vi "TDMS Copy Channel Data.vi"(5 "channel name":string, 7 "group name":string, 8 "error in":errorcluster, 9 "Chunk Size (65536)":i64=65536 min=1, 10 "tdms dest in":refnum<k34>, 11 "tdms source in":refnum<k34>) -> (0 "error out":errorcluster, 2 "tdms dest out":refnum<k34>, 3 "tdms source out":refnum<k34>)   [LabVIEW 2011]
doc: "Copies the data from Channel in the source file to the destintion file. If the channel exists there, the data is appended to the old one."
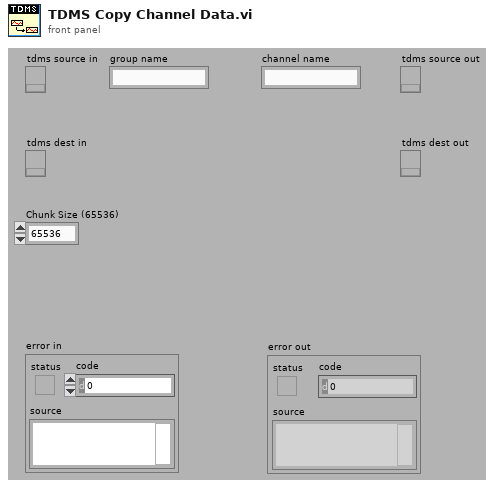
[diagram p1: front panel]
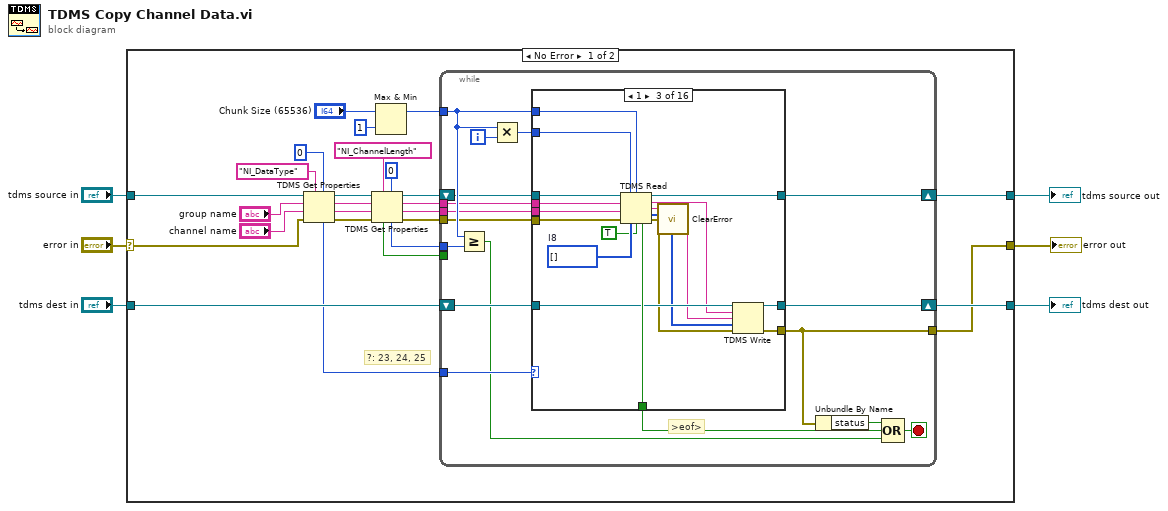
[diagram p0: block diagram]
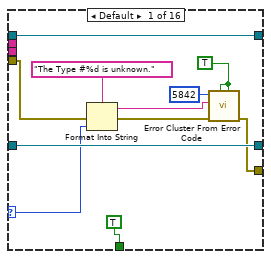
[diagram p2: hidden frame]
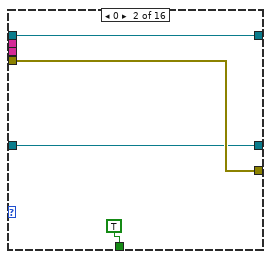
[diagram p3: hidden frame]
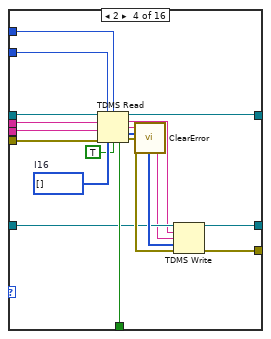
[diagram p4: hidden frame]
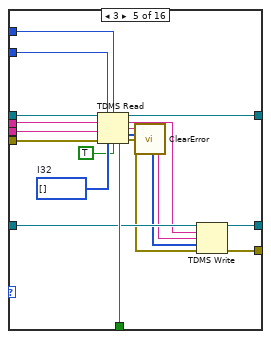
[diagram p5: hidden frame]
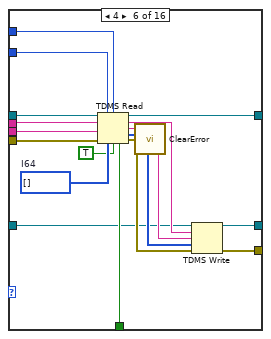
[diagram p6: hidden frame]
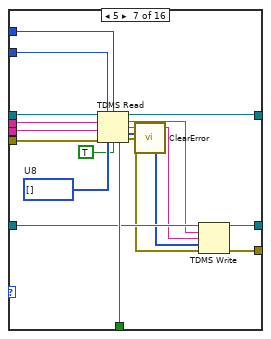
[diagram p7: hidden frame]
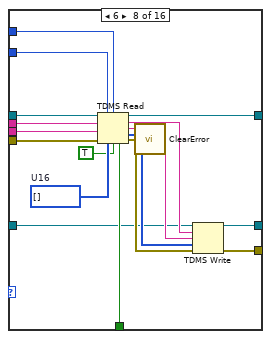
[diagram p8: hidden frame]
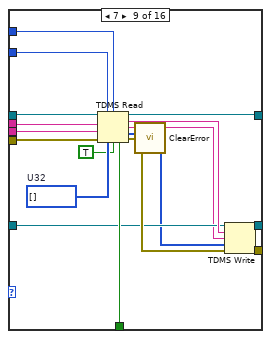
[diagram p9: hidden frame]
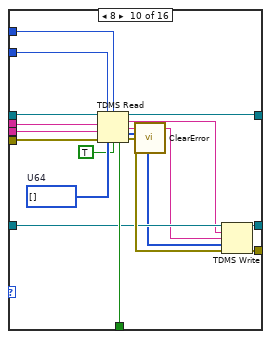
[diagram p10: hidden frame]
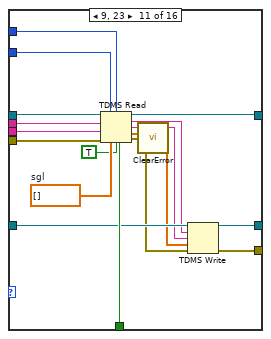
[diagram p11: hidden frame]
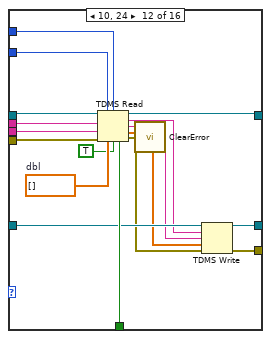
[diagram p12: hidden frame]
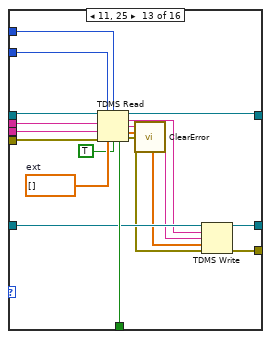
[diagram p13: hidden frame]
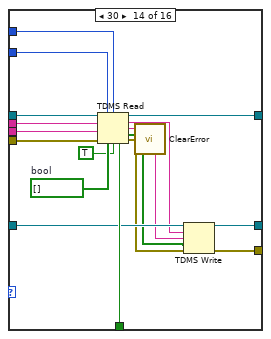
[diagram p14: hidden frame]
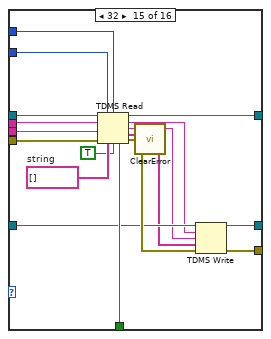
[diagram p15: hidden frame]
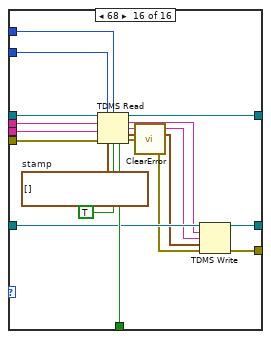
[diagram p16: hidden frame]
diagram:
  n1 = case shown="No Error" "error in" {
    selector: "error in" -> [w7 w319]
    tunnel: "tdms dest in" -> [w24 w318]
    tunnel: [w23 w318] -> w5
    tunnel: [w22 w319] -> w4
    tunnel: [w21 w317] -> w3
    tunnel: "tdms source in" -> [w13 w317]
    frame No Error {
      # "?: 23, 24, 25"
      n2 = TDMS Get Properties(5:0, 7:"NI_DataType" ("property name"), 8:w7, 9:"channel name", 10:"group name", 11:w13) -> (0:w18:errorcluster, 1:w17:string, 2:w16:string, 3:w15:refnum<k34>, 4:w14:i32)  [unwired: 1 out]
      n3 = TDMS Get Properties(5:i64 0, 7:"NI_ChannelLength" ("property name"), 8:w18, 9:w17, 10:w16, 11:w15) -> (0:w27:errorcluster, 1:w28:string, 2:w29:string, 3:w30:refnum<k34>, 4:w26:i64, 6:w25:bool)
      n4 = Max & Min(x="Chunk Size (65536)", y=i64 1) -> (max(x,y)=w10:i64)  [unwired: 1 out]
      n5 = while {
        tunnel: w28 -> [w44]
        tunnel: w27 -> [w43]
        shift-right: [w42] -> w21
        shift-left: w30 -> [w46]
        tunnel: w10 -> [w49]
        tunnel: [w48] -> w22
        tunnel: w14 -> [w40]
        tunnel: w26 -> [w37]
        tunnel: w25 -> [_]
        shift-right: [w35] -> w23
        shift-left: w24 -> [w47]
        tunnel: w29 -> [w45]
        i -> [w34]
        stop <- w33 stop-if-true
        # ">eof>"
        n6 = Greater Or Equal?(x=w49, y=w37) -> (x >= y?=w36:bool)
        n7 = Multiply(x=w49, y=w34) -> (x*y=w41:i64)
        n8 = case shown="1" w40 {
          selector: w40 -> [w52 _ _ _ _ _ _ _ _ _ _ _ _ _ _ _]
          tunnel: w47 -> [w58 w61 w73 w87 w109 w122 w145 w158 w179 w198 w217 w233 w251 w271 w287 w307]
          tunnel: w46 -> [w60 w64 w82 w100 w118 w136 w154 w172 w190 w208 w226 w244 w262 w280 w298 w316]
          tunnel: w45 -> [_ _ w81 w99 w116 w135 w151 w170 w188 w206 w224 w242 w260 w278 w296 w315]
          tunnel: w44 -> [_ _ w80 w98 w115 w134 w150 w169 w187 w205 w223 w241 w259 w277 w291 w314]
          tunnel: w43 -> [w54 w62 w79 w96 w114 w133 w149 w168 w189 w207 w225 w240 w258 w272 w295 w309]
          tunnel: [w60 w64 w77 w97 w117 w131 w153 w171 w185 w203 w222 w243 w261 w279 w297 w313] -> w42
          tunnel: w41 -> [_ _ w75 w93 w110 w129 w146 w165 w183 w201 w219 w238 w256 w274 w292 w311]
          tunnel: w49 -> [_ _ w76 w92 w111 w130 w147 w166 w184 w202 w220 w239 w257 w275 w293 w312]
          tunnel: [w57 w62 w71 w90 w107 w126 w143 w163 w175 w194 w211 w235 w253 w265 w288 w305] -> w48
          tunnel: [TRUE ("eof") TRUE ("eof") w74 w95 w113 w128 w152 w167 w186 w204 w221 w237 w255 w276 w294 w310] -> w38
          tunnel: [w58 w61 w67 w89 w108 w121 w142 w157 w176 w193 w212 w234 w252 w266 w286 w304] -> w35
          frame Default {
            w50 = TRUE ("is warning? (False)")
            n9 = Format Into String(format string="The Type #%d is unknown." ("Format-String"), error in=w54, w52) -> (resulting string=w55:string, error out=w53:errorcluster)  [unwired: 1 in]
            n10 = call <vilib>:"Error Cluster From Error Code.vi"("is warning? (False)"=w50, "show call chain? (False)"=w50, "error in (no error)"=w53, "error message (\"\")"=w55, "error code (0)"=5842) -> ("error out"=w57:errorcluster)  [unwired: 4 out]
          }
          frame 0 {
          }
          frame 1 {
            w78 = i8[] []  # I8
            n11 = TDMS Read(0:w82, 1:w75, 2:w76, 5:w81, 7:w80, 11:w79, 12:w78, 13:TRUE ("return channels in file order? (F)")) -> (4:w77:refnum<k34>, 6:w68:string, 8:w69:string, 10:w70:i8[], 14:w74:bool, 15:w66:errorcluster)
            n12 = call <vilib>:"ClearError.vi"("error in (no error)"=w66) -> ("error out"=w72:errorcluster)
            n13 = TDMS Write(0:w73, 5:w68, 7:w69, 9:w70, 11:w72) -> (4:w67:refnum<k34>, 15:w71:errorcluster)  [unwired: 1 in, 2 out]
          }
          frame 2 {
            w94 = i16[] []  # I16
            n14 = TDMS Read(0:w100, 1:w93, 2:w92, 5:w99, 7:w98, 11:w96, 12:w94, 13:TRUE ("return channels in file order? (F)")) -> (4:w97:refnum<k34>, 6:w86:string, 8:w85:string, 10:w88:i16[], 14:w95:bool, 15:w84:errorcluster)
            n15 = call <vilib>:"ClearError.vi"("error in (no error)"=w84) -> ("error out"=w91:errorcluster)
            n16 = TDMS Write(0:w87, 5:w86, 7:w85, 9:w88, 11:w91) -> (4:w89:refnum<k34>, 15:w90:errorcluster)  [unwired: 1 in, 2 out]
          }
          frame 3 {
            w112 = i32[] []  # I32
            n17 = TDMS Read(0:w118, 1:w110, 2:w111, 5:w116, 7:w115, 11:w114, 12:w112, 13:TRUE ("return channels in file order? (F)")) -> (4:w117:refnum<k34>, 6:w103:string, 8:w105:string, 10:w104:i32[], 14:w113:bool, 15:w102:errorcluster)
            n18 = call <vilib>:"ClearError.vi"("error in (no error)"=w102) -> ("error out"=w106:errorcluster)
            n19 = TDMS Write(0:w109, 5:w103, 7:w105, 9:w104, 11:w106) -> (4:w108:refnum<k34>, 15:w107:errorcluster)  [unwired: 1 in, 2 out]
          }
          frame 4 {
            w132 = i64[] []  # I64
            n20 = TDMS Read(0:w136, 1:w129, 2:w130, 5:w135, 7:w134, 11:w133, 12:w132, 13:TRUE ("return channels in file order? (F)")) -> (4:w131:refnum<k34>, 6:w123:string, 8:w124:string, 10:w125:i64[], 14:w128:bool, 15:w120:errorcluster)
            n21 = call <vilib>:"ClearError.vi"("error in (no error)"=w120) -> ("error out"=w127:errorcluster)
            n22 = TDMS Write(0:w122, 5:w123, 7:w124, 9:w125, 11:w127) -> (4:w121:refnum<k34>, 15:w126:errorcluster)  [unwired: 1 in, 2 out]
          }
          frame 5 {
            w148 = u8[] []  # U8
            n23 = TDMS Read(0:w154, 1:w146, 2:w147, 5:w151, 7:w150, 11:w149, 12:w148, 13:TRUE ("return channels in file order? (F)")) -> (4:w153:refnum<k34>, 6:w139:string, 8:w140:string, 10:w141:u8[], 14:w152:bool, 15:w138:errorcluster)
            n24 = call <vilib>:"ClearError.vi"("error in (no error)"=w138) -> ("error out"=w144:errorcluster)
            n25 = TDMS Write(0:w145, 5:w139, 7:w140, 9:w141, 11:w144) -> (4:w142:refnum<k34>, 15:w143:errorcluster)  [unwired: 1 in, 2 out]
          }
          frame 6 {
            w164 = u16[] []  # U16
            n26 = TDMS Read(0:w172, 1:w165, 2:w166, 5:w170, 7:w169, 11:w168, 12:w164, 13:TRUE ("return channels in file order? (F)")) -> (4:w171:refnum<k34>, 6:w159:string, 8:w160:string, 10:w161:u16[], 14:w167:bool, 15:w156:errorcluster)
            n27 = call <vilib>:"ClearError.vi"("error in (no error)"=w156) -> ("error out"=w162:errorcluster)
            n28 = TDMS Write(0:w158, 5:w159, 7:w160, 9:w161, 11:w162) -> (4:w157:refnum<k34>, 15:w163:errorcluster)  [unwired: 1 in, 2 out]
          }
          frame 7 {
            w182 = u32[] []  # U32
            n29 = TDMS Read(0:w190, 1:w183, 2:w184, 5:w188, 7:w187, 11:w189, 12:w182, 13:TRUE ("return channels in file order? (F)")) -> (4:w185:refnum<k34>, 6:w180:string, 8:w178:string, 10:w177:u32[], 14:w186:bool, 15:w174:errorcluster)
            n30 = call <vilib>:"ClearError.vi"("error in (no error)"=w174) -> ("error out"=w181:errorcluster)
            n31 = TDMS Write(0:w179, 5:w180, 7:w178, 9:w177, 11:w181) -> (4:w176:refnum<k34>, 15:w175:errorcluster)  [unwired: 1 in, 2 out]
          }
          frame 8 {
            w200 = u64[] []  # U64
            n32 = TDMS Read(0:w208, 1:w201, 2:w202, 5:w206, 7:w205, 11:w207, 12:w200, 13:TRUE ("return channels in file order? (F)")) -> (4:w203:refnum<k34>, 6:w195:string, 8:w196:string, 10:w197:u64[], 14:w204:bool, 15:w192:errorcluster)
            n33 = call <vilib>:"ClearError.vi"("error in (no error)"=w192) -> ("error out"=w199:errorcluster)
            n34 = TDMS Write(0:w198, 5:w195, 7:w196, 9:w197, 11:w199) -> (4:w193:refnum<k34>, 15:w194:errorcluster)  [unwired: 1 in, 2 out]
          }
          frame 9, 23 {
            w218 = sgl[] []  # sgl
            n35 = TDMS Read(0:w226, 1:w219, 2:w220, 5:w224, 7:w223, 11:w225, 12:w218, 13:TRUE ("return channels in file order? (F)")) -> (4:w222:refnum<k34>, 6:w215:string, 8:w214:string, 10:w213:sgl[], 14:w221:bool, 15:w210:errorcluster)
            n36 = call <vilib>:"ClearError.vi"("error in (no error)"=w210) -> ("error out"=w216:errorcluster)
            n37 = TDMS Write(0:w217, 5:w215, 7:w214, 9:w213, 11:w216) -> (4:w212:refnum<k34>, 15:w211:errorcluster)  [unwired: 1 in, 2 out]
          }
          frame 10, 24 {
            w236 = dbl[] []  # dbl
            n38 = TDMS Read(0:w244, 1:w238, 2:w239, 5:w242, 7:w241, 11:w240, 12:w236, 13:TRUE ("return channels in file order? (F)")) -> (4:w243:refnum<k34>, 6:w229:string, 8:w230:string, 10:w232:dbl[], 14:w237:bool, 15:w228:errorcluster)
            n39 = call <vilib>:"ClearError.vi"("error in (no error)"=w228) -> ("error out"=w231:errorcluster)
            n40 = TDMS Write(0:w233, 5:w229, 7:w230, 9:w232, 11:w231) -> (4:w234:refnum<k34>, 15:w235:errorcluster)  [unwired: 1 in, 2 out]
          }
          frame 11, 25 {
            w254 = ext[] []  # ext
            n41 = TDMS Read(0:w262, 1:w256, 2:w257, 5:w260, 7:w259, 11:w258, 12:w254, 13:TRUE ("return channels in file order? (F)")) -> (4:w261:refnum<k34>, 6:w247:string, 8:w248:string, 10:w250:ext[], 14:w255:bool, 15:w246:errorcluster)
            n42 = call <vilib>:"ClearError.vi"("error in (no error)"=w246) -> ("error out"=w249:errorcluster)
            n43 = TDMS Write(0:w251, 5:w247, 7:w248, 9:w250, 11:w249) -> (4:w252:refnum<k34>, 15:w253:errorcluster)  [unwired: 1 in, 2 out]
          }
          frame 30 {
            w273 = bool[] []  # bool
            n44 = TDMS Read(0:w280, 1:w274, 2:w275, 5:w278, 7:w277, 11:w272, 12:w273, 13:TRUE ("return channels in file order? (F)")) -> (4:w279:refnum<k34>, 6:w267:string, 8:w268:string, 10:w269:bool[], 14:w276:bool, 15:w264:errorcluster)
            n45 = call <vilib>:"ClearError.vi"("error in (no error)"=w264) -> ("error out"=w270:errorcluster)
            n46 = TDMS Write(0:w271, 5:w267, 7:w268, 9:w269, 11:w270) -> (4:w266:refnum<k34>, 15:w265:errorcluster)  [unwired: 1 in, 2 out]
          }
          frame 32 {
            w290 = string[] []  # string
            n47 = TDMS Read(0:w298, 1:w292, 2:w293, 5:w296, 7:w291, 11:w295, 12:w290, 13:TRUE ("return channels in file order? (F)")) -> (4:w297:refnum<k34>, 6:w285:string, 8:w284:string, 10:w283:string[], 14:w294:bool, 15:w282:errorcluster)
            n48 = call <vilib>:"ClearError.vi"("error in (no error)"=w282) -> ("error out"=w289:errorcluster)
            n49 = TDMS Write(0:w287, 5:w285, 7:w284, 9:w283, 11:w289) -> (4:w286:refnum<k34>, 15:w288:errorcluster)  [unwired: 1 in, 2 out]
          }
          frame 68 {
            w308 = timestamp[] []  # stamp
            n50 = TDMS Read(0:w316, 1:w311, 2:w312, 5:w315, 7:w314, 11:w309, 12:w308, 13:TRUE ("return channels in file order? (F)")) -> (4:w313:refnum<k34>, 6:w303:string, 8:w302:string, 10:w301:timestamp[], 14:w310:bool, 15:w300:errorcluster)
            n51 = call <vilib>:"ClearError.vi"("error in (no error)"=w300) -> ("error out"=w306:errorcluster)
            n52 = TDMS Write(0:w307, 5:w303, 7:w302, 9:w301, 11:w306) -> (4:w304:refnum<k34>, 15:w305:errorcluster)  [unwired: 1 in, 2 out]
          }
        }
        n53 = Unbundle By Name(w48) -> ("status"=w39:bool)
        n54 = Compound Arithmetic op=OR(w39, w38, w36) -> (w33:bool)
      }
    }
    frame Error {
    }
  }
  "error out" <- w4
  "tdms source out" <- w3
  "tdms dest out" <- w5
